vi "Write Setting.vi"(8 "error in (no error)":errorcluster, 10 "Setting":sgl[](array[numeric]), 11 "Update SGL Array in":refnum<class "Update SGL Array.lvclass">) -> (0 "error out":errorcluster, 3 "Update SGL Array out":refnum<class "Update SGL Array.lvclass">)   [LabVIEW 2014, in "Update SGL Array.lvclass"]
uses:
  Update SGL Array.lvclass
  Update SGL Array.lvclass/Update SGL Array.ctl
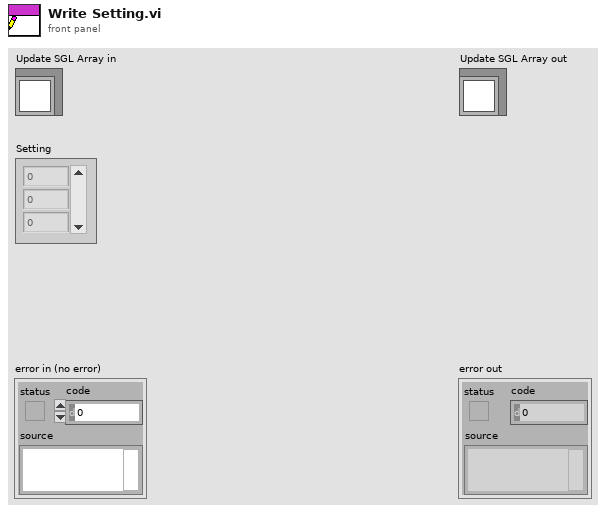
[diagram p1: front panel]
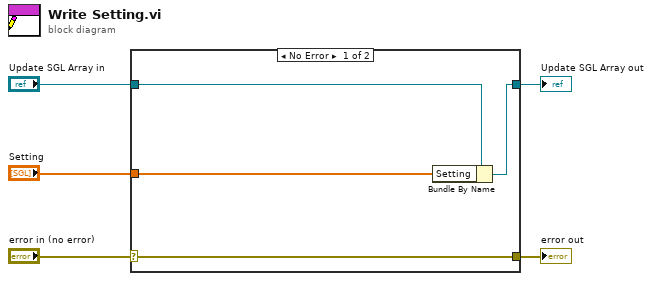
[diagram p0: block diagram]
diagram:
  n1 = case shown="No Error" "error in (no error)" {
    selector: "error in (no error)" -> [w9 w10]
    tunnel: [w9 w10] -> w4
    tunnel: [w7 w11] -> w2
    tunnel: "Update SGL Array in" -> [w8 w11]
    tunnel: "Setting" -> [w6 _]
    frame No Error {
      n2 = Bundle By Name(cluster=w8, "Setting"=w6) -> (w7:refnum<class "Update SGL Array.lvclass">)
    }
    frame Error {
    }
  }
  "error out" <- w4
  "Update SGL Array out" <- w2
